vi "testCustomAssertionFailureMessage.vi"() -> ()   [LabVIEW 2017, in "Assertion.Tests.lvlib" / "AssertErrorCode.lvlib"]
uses:
  AssertErrorCode.lvlib
  <vilib>/Utility/error.llb/Error Cluster From Error Code.vi
  <vilib>/ErrorRing/Error Ring.xnode
  Assertion/Assertion.lvlib
panel:
  out "error out":errorcluster
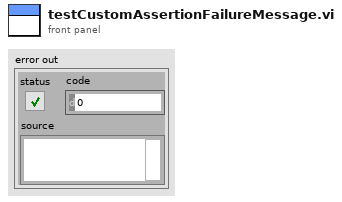
[diagram p1: front panel]
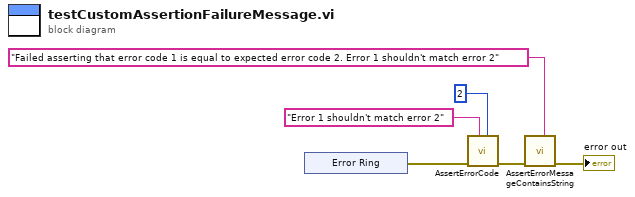
[diagram p0: block diagram]
diagram:
  n1 = xnode "Error Ring"() -> ("error out"=w6:errorcluster)
  n2 = call "AssertErrorCode.vi"("Expected"=2, "Message (\"\")"="Error 1 shouldn't match error 2" ("Message (\"\")"), "error in (no error)"=w6) -> ("error out"=w1:errorcluster)  [unwired: 8 in]
  n3 = call "AssertErrorMessageContainsString.vi"("Expected"="Failed asserting that error code 1 is equal to expected error code 2. Error 1 shouldn't match error 2" ("Needle"), "error in (no error)"=w1) -> ("error out"=→"error out":errorcluster)  [unwired: 9 in]
